vi "读标定功率检测值解析.vi"(9 "读取的字节":i32, 10 "响应":string) -> (1 "消息":string, 2 "读标定功率检测值":string[](array[string]))   [LabVIEW 2015]
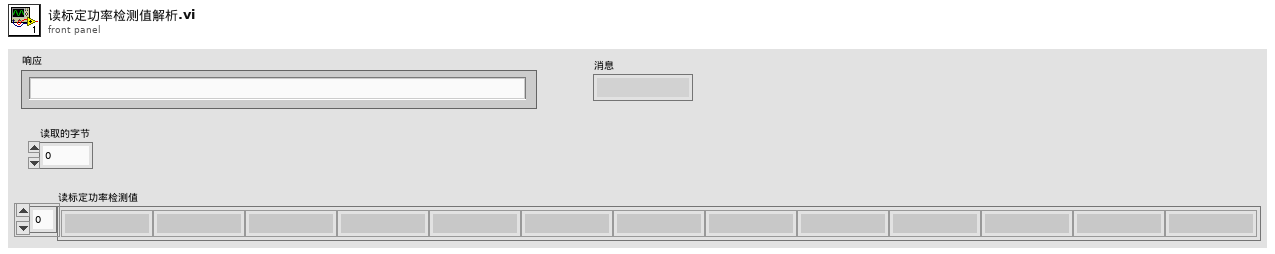
[diagram p1: front panel]
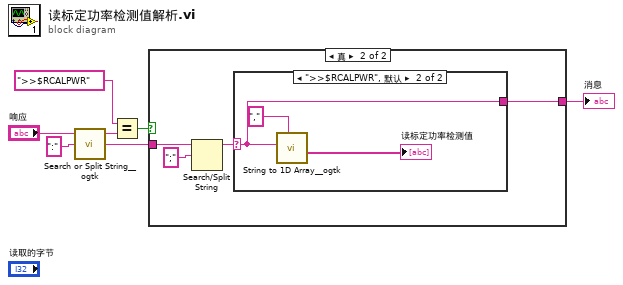
[diagram p0: block diagram]
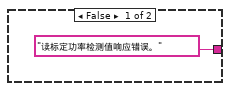
[diagram p2: hidden frame]
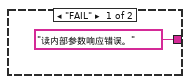
[diagram p3: hidden frame]
diagram:
  n1 = call <userlib>:"Search or Split String__ogtk.vi"("search string/char (-)"=":", "string"="响应") -> ("substring after match"=w2:string, "substring before match"=w5:string)  [unwired: 1 in, 1 out]
  n2 = Equal?(x=">>$RCALPWR" ("消息"), y=w5) -> (x = y?=w3:bool)
  n3 = case shown="真" w3 {
    tunnel: w2 -> [_ w11]
    tunnel: ["读标定功率检测值响应错误。" ("消息") w9] -> w1
    frame False {
    }
    frame True {
      n4 = Search/Split String(string=w11, search string/char (-)=";" ("搜索字符串/字符(-)")) -> (substring before match=w10:string)  [unwired: 1 in, 2 out]
      n5 = case shown="\">>$RCALPWR\", 默认" w10 {
        selector: w10 -> [_ w15]
        tunnel: ["读内部参数响应错误。" ("消息") w15] -> w9
        frame "FAIL" {
        }
        frame ">>$RCALPWR", Default {
          n6 = call <userlib>:"String to 1D Array__ogtk.vi"("delimiter (Tab)"=",", "string"=w15) -> ("Array of Strings"=→"读标定功率检测值":string[])  [unwired: 9 in]
        }
      }
    }
  }
  "消息" <- w1
